vi "Config.File.Read.vi"(8 "error in":errorcluster, 11 "path":path) -> (0 "error out":errorcluster)   [LabVIEW 2016]
uses:
  Tma.lib/nlconfig.llb/fp2ini mode.ctl
  Config.Global.vi
  Global/ApplicationGlobal.vi
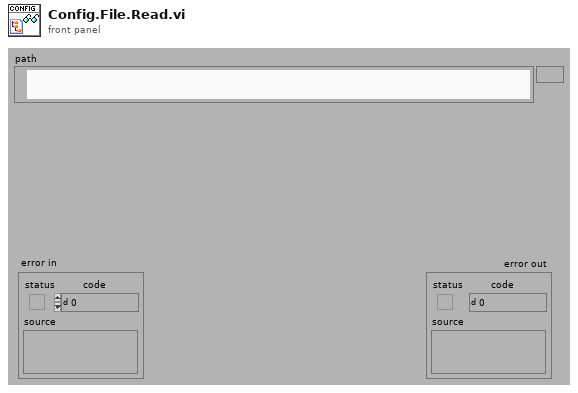
[diagram p1: front panel]
types:
  T1 = typedef "fp2ini mode.ctl" = enum16{"Read Controls", "Write Controls", "Write Indicators", "Read Indicators", "Write all", "Read all"}
  T2 = typedef "Sequence.UserData.ctl" = cluster{"GuiMode":T3, "Test":T4, "ContinueOrder":bool}
  T3 = typedef "Sequence.MainMode.ctl" = enum16{"Process", "Base", "Order", "Manual", "Logs", "Results", "Stats", "DMC Config"}
  T4 = typedef "MainGui.TestOptions.ctl" = cluster{"IgnoreResults":bool, "IgnoreImages":bool, "ServiceMode":bool}
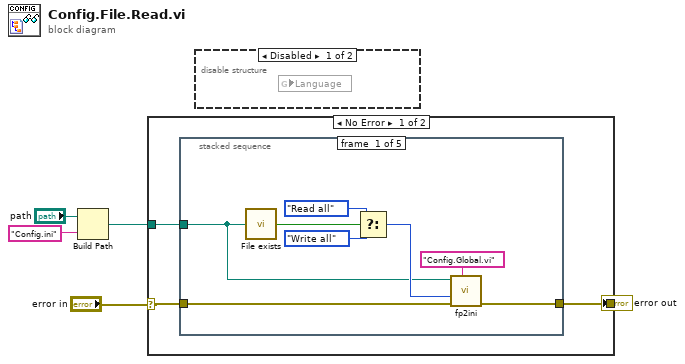
[diagram p0: block diagram]
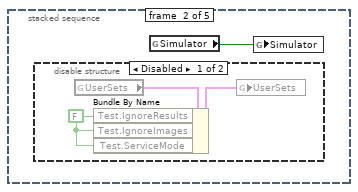
[diagram p3: hidden frame]
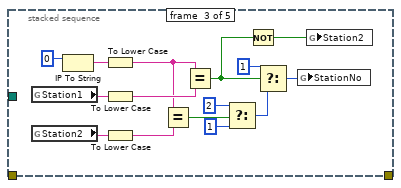
[diagram p5: hidden frame]
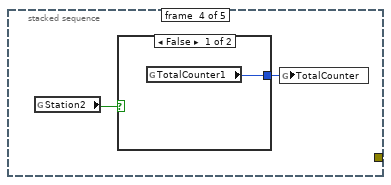
[diagram p6: hidden frame]
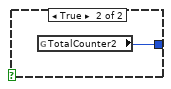
[diagram p7: hidden frame]
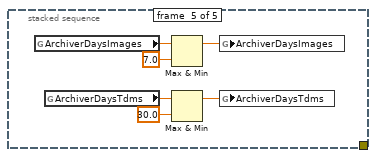
[diagram p8: hidden frame]
diagram:
  n1 = Build Path(base path="path", name or relative path="Config.ini") -> (appended path=w1:path)
  n2 = case shown="No Error" "error in" {
    selector: "error in" -> [w8 w46]
    tunnel: [w7 w46] -> w5
    tunnel: w1 -> [w6 _]
    frame No Error {
      n3 = stacked-sequence {
        tunnel: w8 -> [w16 _ _ _ _]
        tunnel: [w15 _ _ _ _] -> w7
        tunnel: w6 -> [w9 _ _ _ _]
        frame #0 {
          n4 = call "File exists.vi"("file path"=w9) -> ("exists?"=w13:bool)  [unwired: 4 in]
          n5 = Select(t=fp2ini_mode."Read all" ("mode"), s=w13, f=fp2ini_mode."Write all" ("mode")) -> (s? t:f=w11:T1)
          n6 = call "fp2ini.vi"("vi-name (caller if empty)"="Config.Global.vi", "error in"=w16, "mode"=w11, "ini-file path"=w9) -> ("error out"=w15:errorcluster)  [unwired: 7 in]
        }
        frame #1 {
          n7 = disable-structure shown="Disabled" {
            frame Disabled {
              w18 = FALSE ("Auto.IgnoreResults")
              n8 = global read "Config.Global.vi" "UserSets"() -> (w20:T2)
              n9 = Bundle By Name(cluster=w20, "Test.IgnoreResults"=w18, "Test.IgnoreImages"=w18, "Test.ServiceMode"=w18) -> (w19:T2)
              n10 = global write "Config.Global.vi" "UserSets"(w19) -> ()
            }
            frame Enabled {
            }
          }
          n11 = global read "Config.Global.vi" "Simulator"() -> (w17:bool)
          n12 = global write "ApplicationGlobal.vi" "Simulator"(w17) -> ()
        }
        frame #2 {
          n13 = global read "Config.Global.vi" "Station1"() -> (w34:string)
          n14 = global read "Config.Global.vi" "Station2"() -> (w32:string)
          n15 = IP To String(2:u32 0 ("net address")) -> (0:w33:string)  [unwired: 1 in]
          n16 = To Lower Case(string=w33) -> (all lower case string=w30:string)
          n17 = To Lower Case(string=w34) -> (all lower case string=w31:string)
          n18 = To Lower Case(string=w32) -> (all lower case string=w29:string)
          n19 = Equal?(x=w30, y=w29) -> (x = y?=w23:bool)
          n20 = Equal?(x=w30, y=w31) -> (x = y?=w22:bool)
          n21 = Select(t=2 ("StationNo"), s=w23, f=1 ("StationNo")) -> (s? t:f=w25:i32)
          n22 = Not(x=w22) -> (.not. x?=w21:bool)
          n23 = Select(t=1 ("StationNo"), s=w22, f=w25) -> (s? t:f=w24:i32)
          n24 = global write "ApplicationGlobal.vi" "StationNo"(w24) -> ()
          n25 = global write "ApplicationGlobal.vi" "Station2"(w21) -> ()
        }
        frame #3 {
          n26 = global read "ApplicationGlobal.vi" "Station2"() -> (w36:bool)
          n27 = case shown="False" w36 {
            tunnel: [w38 w39] -> w37
            frame False {
              n28 = global read "Config.Global.vi" "TotalCounter1"() -> (w38:u32)
            }
            frame True {
              n29 = global read "Config.Global.vi" "TotalCounter2"() -> (w39:u32)
            }
          }
          n30 = global write "ApplicationGlobal.vi" "TotalCounter"(w37) -> ()
        }
        frame #4 {
          n31 = global read "Config.Global.vi" "ArchiverDaysImages"() -> (w45:dbl)
          n32 = global read "Config.Global.vi" "ArchiverDaysTdms"() -> (w40:dbl)
          n33 = Max & Min(x=w45, y=7.0 ("lower limit")) -> (max(x,y)=w43:dbl)  [unwired: 1 out]
          n34 = Max & Min(x=w40, y=30.0 ("lower limit")) -> (max(x,y)=w42:dbl)  [unwired: 1 out]
          n35 = global write "Config.Global.vi" "ArchiverDaysImages"(w43) -> ()
          n36 = global write "Config.Global.vi" "ArchiverDaysTdms"(w42) -> ()
        }
      }
    }
    frame Error {
    }
  }
  "error out" <- w5
  n37 = disable-structure shown="Disabled" {
    frame Disabled {
      n38 = global read "Config.Global.vi" "Language"() -> ()  [unwired: 1 in]
    }
    frame Enabled {
    }
  }
